vi "상태머신.vi"() -> ()   [LabVIEW 2014]
uses:
  <vilib>/Analysis/NI_AALBase.lvlib
panel:
  out "웨이브폼 그래프":dbl[](graph)
  in  "정지":bool
  in  "삼각":bool
  in  "sine":bool
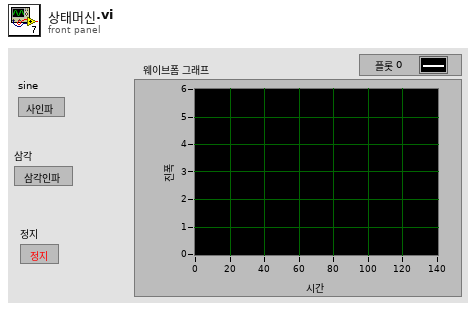
[diagram p1: front panel]
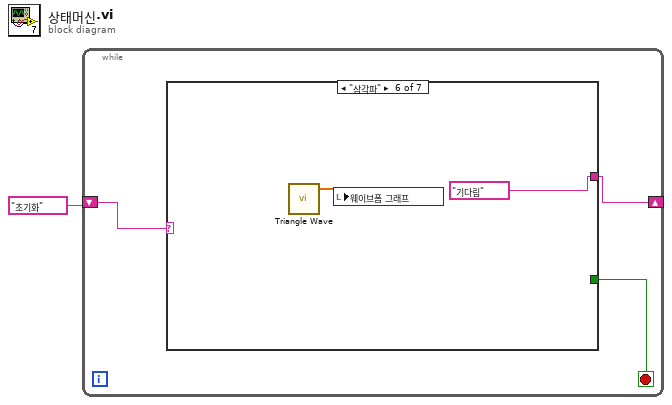
[diagram p0: block diagram]
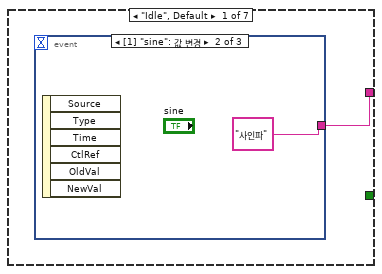
[diagram p2: hidden frame]
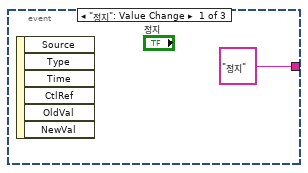
[diagram p3: hidden frame]
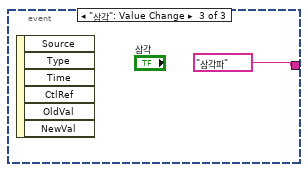
[diagram p4: hidden frame]
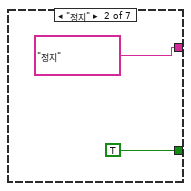
[diagram p5: hidden frame]
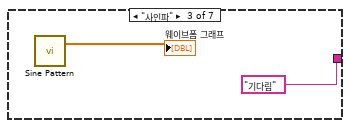
[diagram p6: hidden frame]
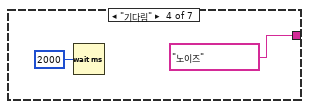
[diagram p7: hidden frame]
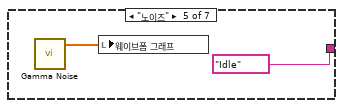
[diagram p8: hidden frame]
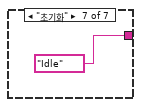
[diagram p9: hidden frame]
diagram:
  n1 = while {
    shift-right: [w2] -> _
    shift-left: "초기화" -> [w3]
    stop <- w4 stop-if-true
    n2 = case shown="\"삼각파\"" w3 {
      tunnel: [w5 "정지" "기다림" "노이즈" "Idle" "기다림" "Idle"] -> w2
      tunnel: [_ TRUE _ _ _ _ _] -> w4
      frame "Idle", Default {
        n3 = event shown="[1] \"sine\": 값 변경" {
          selector: _ -> [_ _ _]
          dyn-events: _ -> [_ _ _]
          timeout: _ -> [_ _ _]
          tunnel: ["정지" "사인파" "삼각파"] -> w5
          event "정지": Value Change {
            n4 = event-data() -> ()  [unwired: 1 in, 6 out]
          }
          event "sine": Value Change {
            n5 = event-data() -> ()  [unwired: 1 in, 6 out]
          }
          event "삼각": Value Change {
            n6 = event-data() -> ()  [unwired: 1 in, 6 out]
          }
        }
      }
      frame "정지" {
      }
      frame "사인파" {
        n7 = call <vilib>:"Sine Pattern.vi"() -> ("Sinusoidal Pattern"=→"웨이브폼 그래프":dbl[])  [unwired: 4 in, 1 out]
      }
      frame "기다림" {
        n8 = Wait (ms)(milliseconds to wait=u32 2000 ("대기 시간(ms)")) -> ()  [unwired: 1 out]
      }
      frame "노이즈" {
        n9 = call <vilib>:"Gamma Noise.vi"() -> ("gamma noise"=w15:dbl[])  [unwired: 10 in, 1 out]
        n10 = local write "웨이브폼 그래프"(w15) -> ()
      }
      frame "삼각파" {
        n11 = call <vilib>:"Triangle Wave.vi"() -> ("triangle wave"=w17:dbl[])  [unwired: 5 in, 2 out]
        n12 = local write "웨이브폼 그래프"(w17) -> ()
      }
      frame "초기화" {
      }
    }
  }
